vi "Scalar Create.vi"   [LabVIEW 2012, in "MDSplus.lvlib"]
uses:
  <vilib>/MDSplus/Library/MDSplus.lvlib
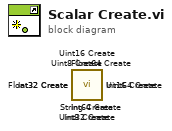
[diagram p0: block diagram]
diagram:
  n1 = call <vilib>:"String Create.vi"() -> ()  [unwired: 10 in, 2 out]
  n2 = call <vilib>:"Float64 Create.vi"() -> ()  [unwired: 10 in, 2 out]
  n3 = call <vilib>:"Float32 Create.vi"() -> ()  [unwired: 10 in, 2 out]
  n4 = call <vilib>:"Uint64 Create.vi"() -> ()  [unwired: 10 in, 2 out]
  n5 = call <vilib>:"Uint32 Create.vi"() -> ()  [unwired: 10 in, 2 out]
  n6 = call <vilib>:"Uint16 Create.vi"() -> ()  [unwired: 10 in, 2 out]
  n7 = call <vilib>:"Uint8 Create.vi"() -> ()  [unwired: 10 in, 2 out]
  n8 = call <vilib>:"Int64 Create.vi"() -> ()  [unwired: 10 in, 2 out]
  n9 = call <vilib>:"Int32 Create.vi"() -> ()  [unwired: 10 in, 2 out]
  n10 = call <vilib>:"Int16 Create.vi"() -> ()  [unwired: 10 in, 2 out]
  n11 = call <vilib>:"Int8 Create.vi"() -> ()  [unwired: 10 in, 2 out]
